vi "Copy start datum.vi"(1 "bytestream":refnum<class "Bytestream.lvclass">) -> (0 "data":u8[](array[numeric]) format="%02x")   [LabVIEW 2020, in "NI_Bytestream.lvlib" / "Bytestream.lvclass"]
uses:
  <vilib>/Array/Bytestream/Bytestream.lvclass
  <vilib>/Array/Bytestream/Bytestream.lvclass/Bytestream.ctl
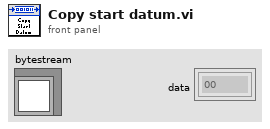
[diagram p1: front panel]
types:
  T1 = typedef "NI_Bytestream.lvlib/Bytestream.lvclass/Datum.ctl" = cluster{"array":u8[], "index":i32}
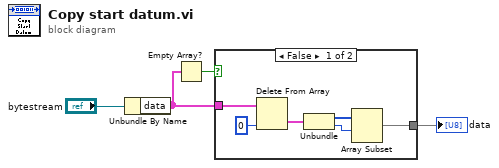
[diagram p0: block diagram]
diagram:
  n1 = Unbundle By Name("bytestream") -> ("data"=w2:T1[])
  n2 = Empty Array?(array=w2) -> (empty?=w1:bool)
  n3 = case shown="False" w1 {
    tunnel: [w10 _] -> w3
    tunnel: w2 -> [w5 _]
    frame False {
      n4 = Delete From Array(array=w5, index=0) -> (deleted portion=w8:T1)  [unwired: 1 in, 1 out]
      n5 = Unbundle(w8) -> ("array"=w7:u8[], "index"=w6:i32)
      n6 = Array Subset(array=w7, index=w6) -> (w10:u8[])  [unwired: 1 in]
    }
    frame True {
    }
  }
  "data" <- w3
